vi "Process.vi"(8 "error in":errorcluster, 11 "demoForJoe":refnum<class "demoForJoe.lvclass">) -> (0 "error out":errorcluster, 3 "demoForJoe out":refnum<class "demoForJoe.lvclass">)   [LabVIEW 2016, in "demoForJoe.lvclass"]
doc: "---------------------------------------------------------------\nJKI State Machine Objects™\nhttp://jki.net/state-machine-objects/\nCopyright (C) 2005-2015, JKI <info@jki.net>\nALL RIGHTS RESERVED"
uses:
  demoForJoe.lvclass
  C:/Program Files (x86)/National Instruments/LabVIEW 2016/vi.lib/JKI/JKI SMO/SMO/SMO.lvclass
  Typedefs/PrivateEvents--demoForJoe.StringMethod.ctl
  <vilib>/JKI/JKI SMO/SMO/Typedefs/Parent Call--Enum.ctl
  <vilib>/JKI/JKI SMO/SMO/SMO.lvclass
panel:
  out "StringMethod":T1
  # "For instructions on how to use the JKI State Machine Objects, examples and video tutorials, visit:\nhttp://jki.net/state-machine-objects/\n\nJKI State Machine Objects™\nhttp://jki.net/state-machine-objects/\nCopyright (C) 2005-2015, JKI <info@jki.net>\nALL RIGHTS RESERVED"
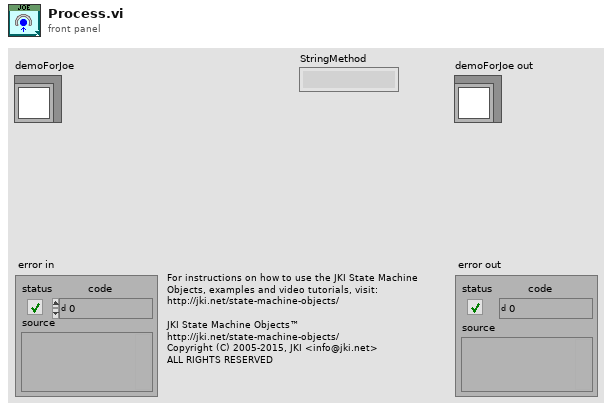
[diagram p1: front panel]
types:
  T1 = typedef "demoForJoe.lvclass/PrivateEvents--demoForJoe.StringMethod.ctl" = string
  T2 = typedef "SMO.lvclass/Parent Call--Enum.ctl" = enum16{"Allows parent to run", "Does not request parent to run"}
  T3 = enum32{"invalid app kind", "Development System", "Run Time System", "Student Edition", "Embedded LabVIEW", "Evaluation", "Custom"}
  T4 = enum32{"Invalid", "Standard", "Closed", "Hidden", "Minimized", "Maximized"}
  T5 = enum32{"Bad", "Idle", "Run top level", "Running"}
  T6 = cluster{"Core":cluster{"Current VI Reference":refnum<vi>, "Close Panel on Exit?":bool, "error":errorcluster}, "Self Reference":refnum<class "demoForJoe.lvclass">, "Your string data":string}
  T7 = cluster{"Current VI Reference":refnum<vi>, "Close Panel on Exit?":bool, "error":errorcluster}
  T8 = typedef "SMO.lvclass/Protected Events.ctl" = cluster{"StopProcesses":refnum<user-event>, "AbortProcesses":refnum<user-event>, "Config Changed":refnum<user-event>, "Dependency":refnum<user-event>}
  T9 = typedef "demoForJoe.lvclass/PrivateEvents--Cluster.ctl" = cluster{"StringMethod":refnum<user-event>}
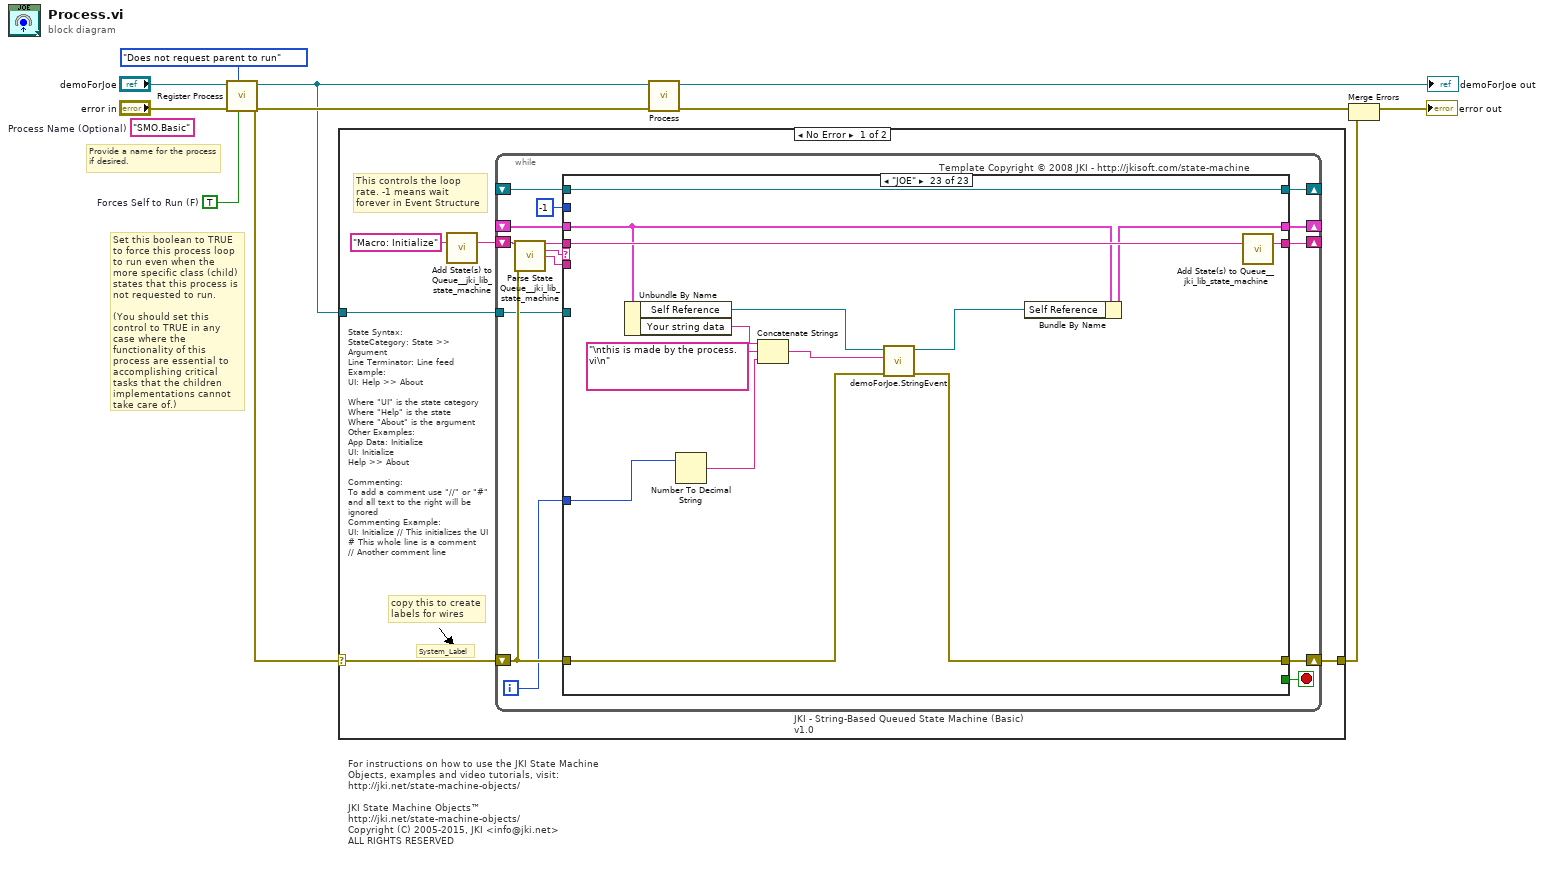
[diagram p0: block diagram]
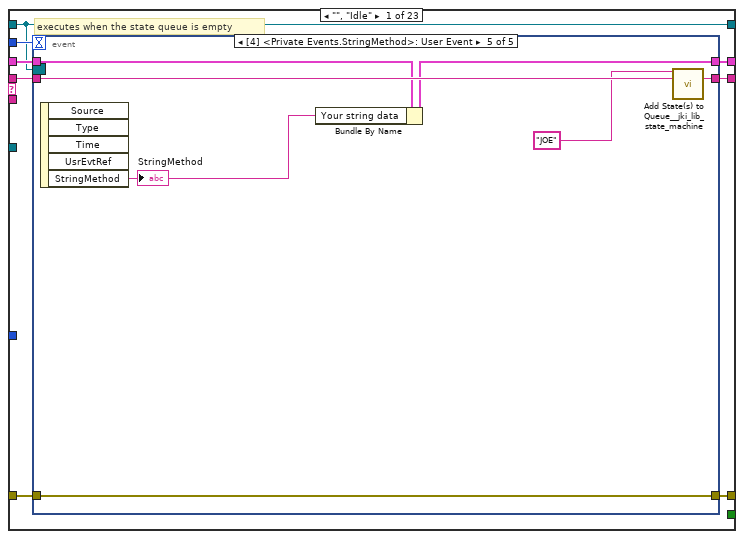
[diagram p2: hidden frame]
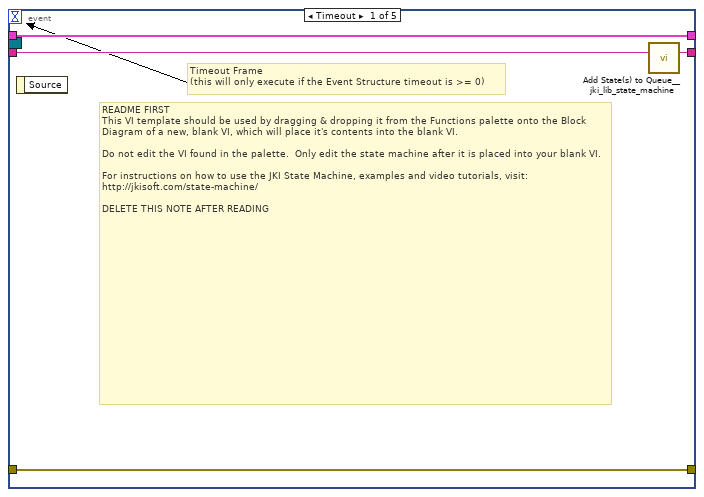
[diagram p3: hidden frame]
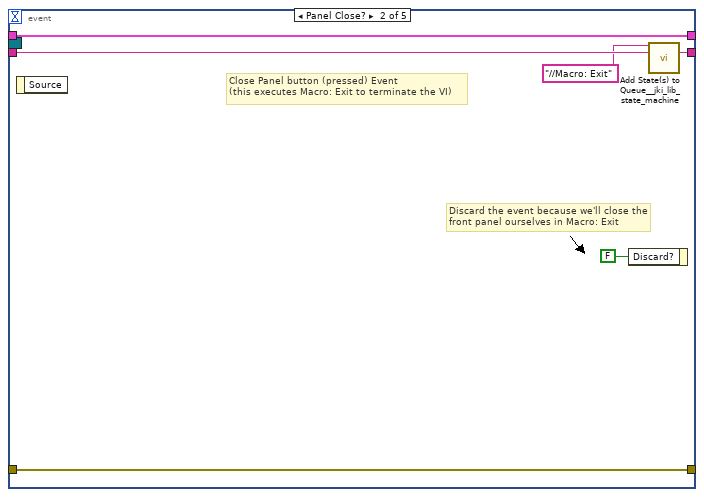
[diagram p4: hidden frame]
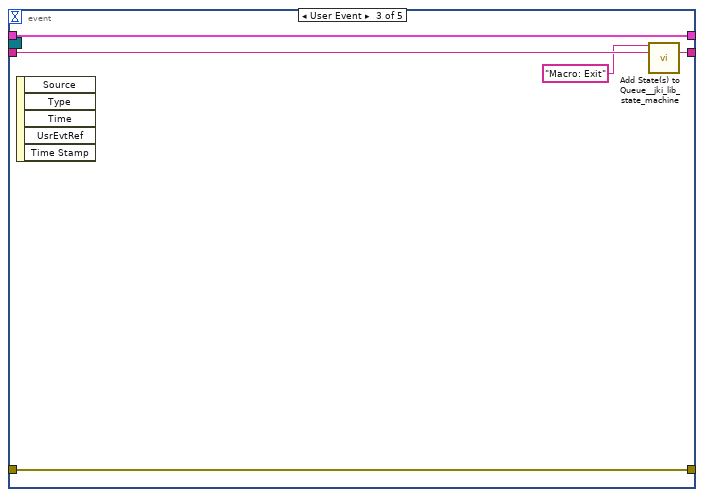
[diagram p5: hidden frame]
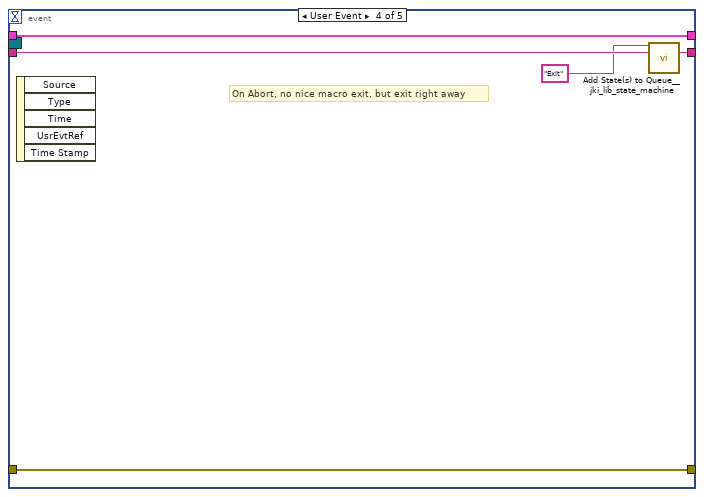
[diagram p6: hidden frame]
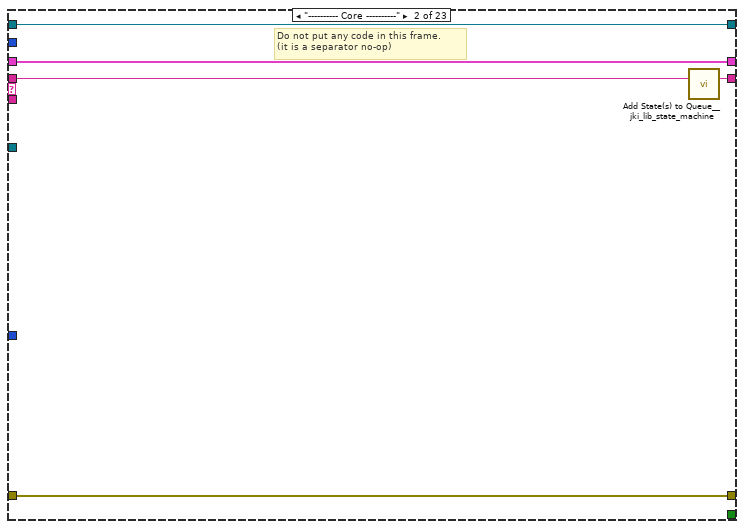
[diagram p7: hidden frame]
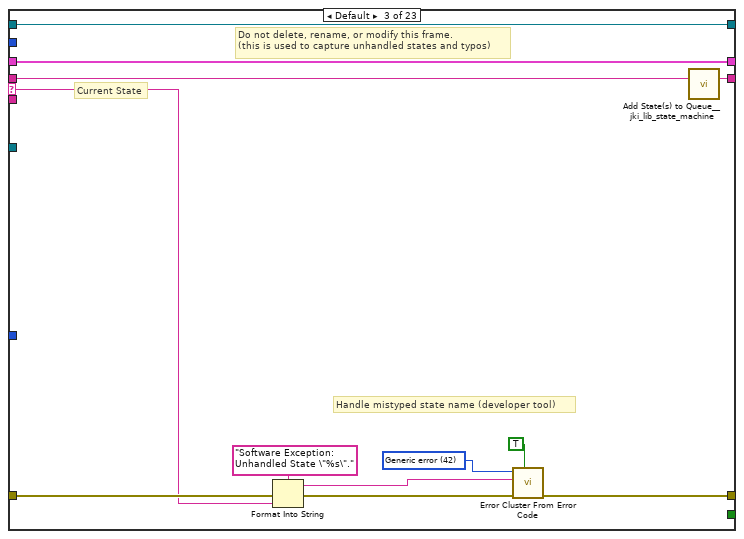
[diagram p8: hidden frame]
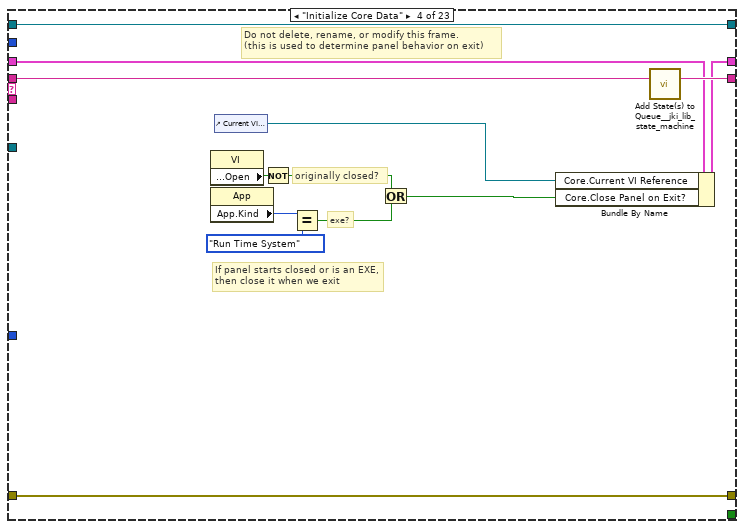
[diagram p9: hidden frame]
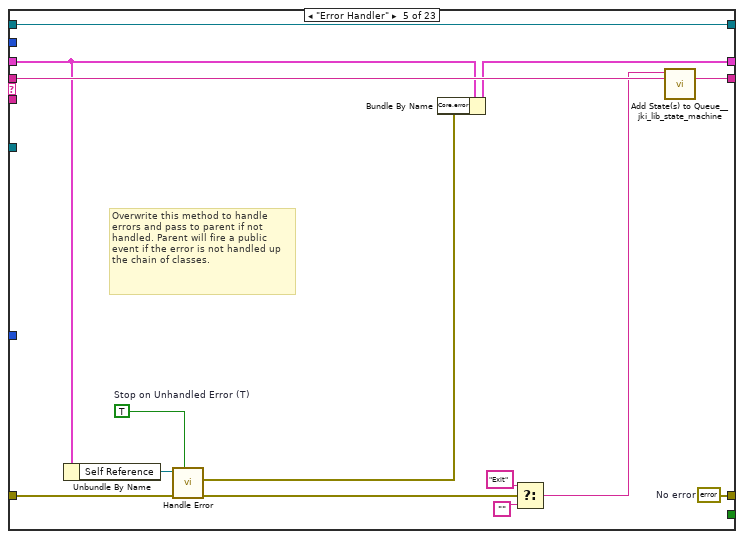
[diagram p10: hidden frame]
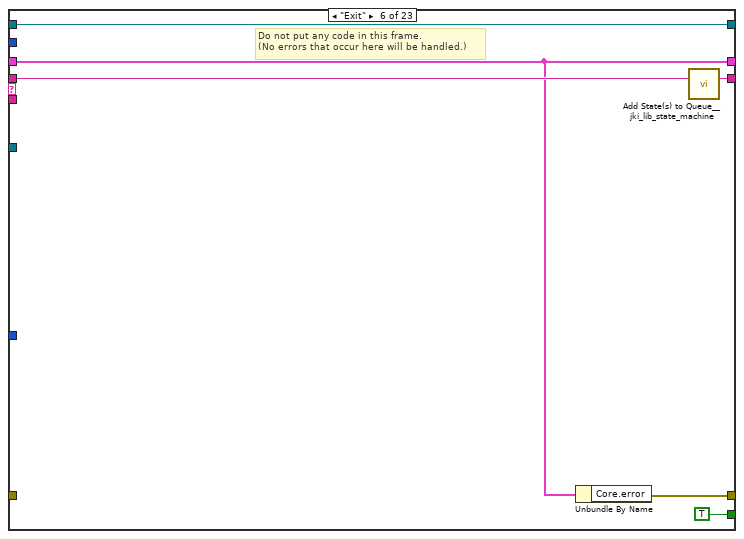
[diagram p11: hidden frame]
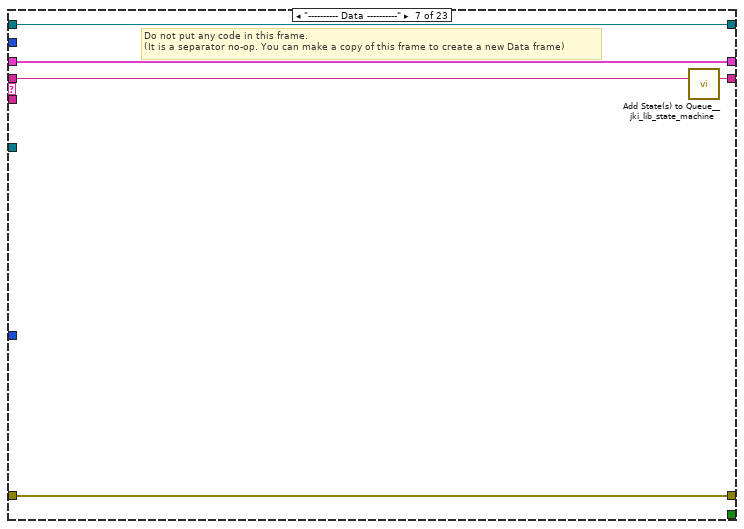
[diagram p12: hidden frame]
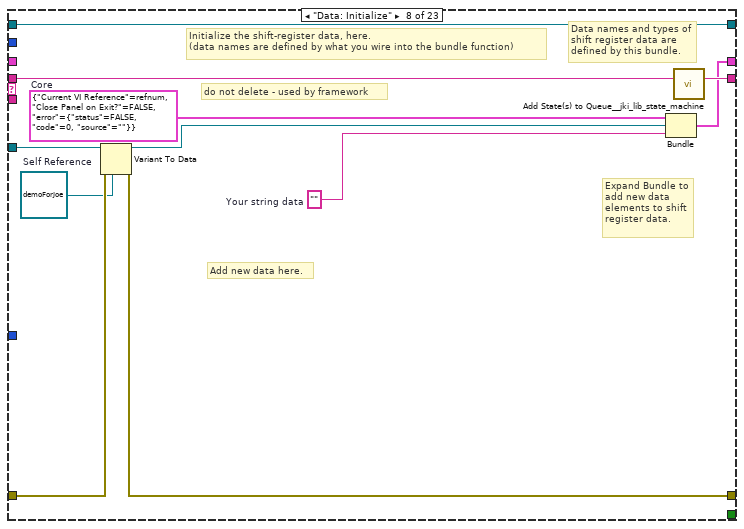
[diagram p13: hidden frame]
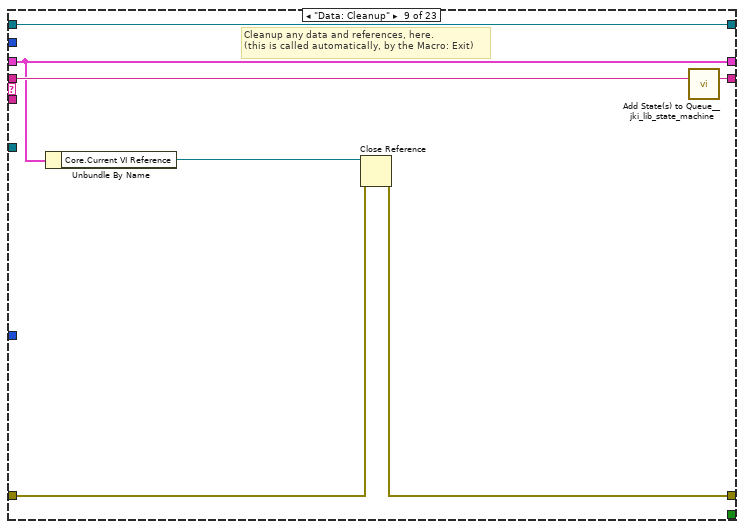
[diagram p14: hidden frame]
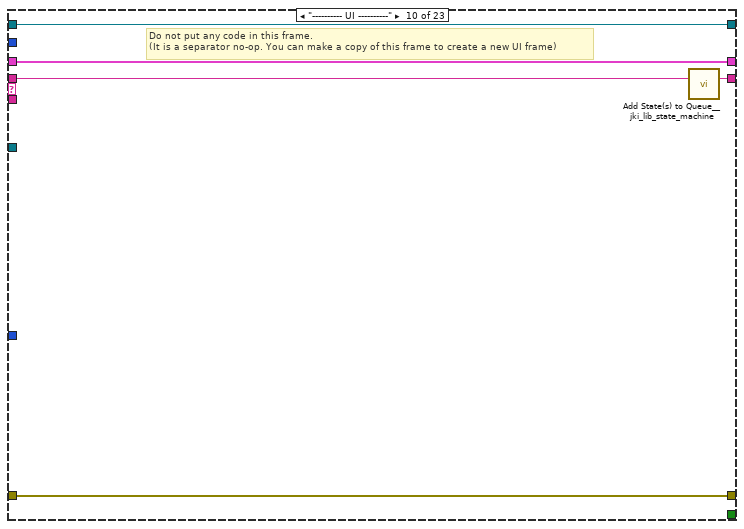
[diagram p15: hidden frame]
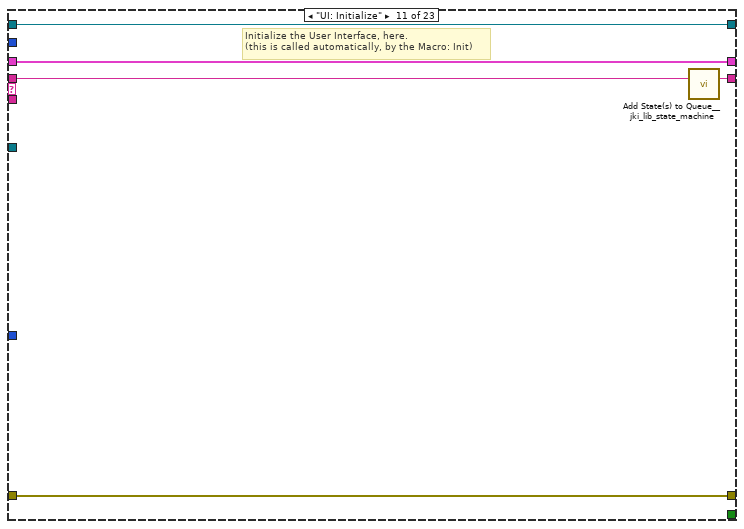
[diagram p16: hidden frame]
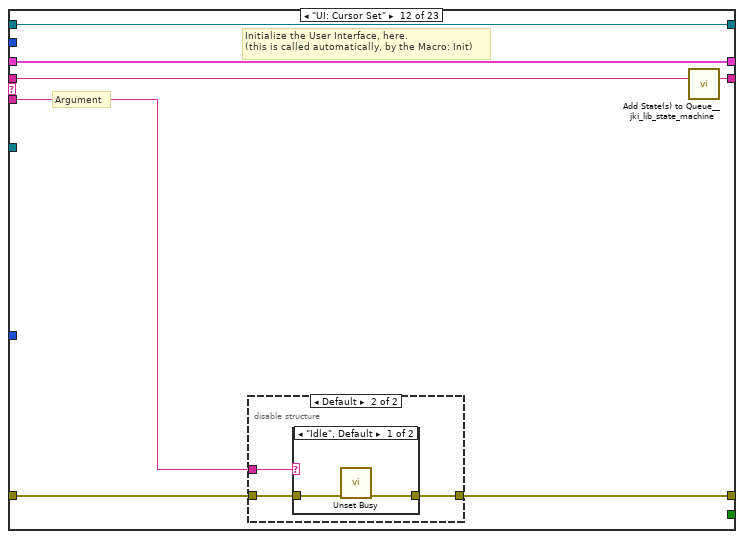
[diagram p17: hidden frame]
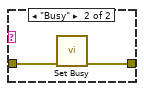
[diagram p19: hidden frame]
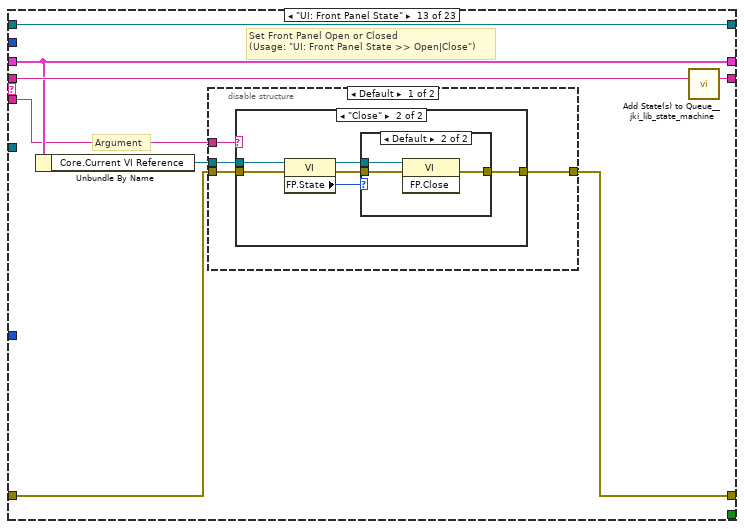
[diagram p20: hidden frame]
diagram:
  w1 = TRUE  # Forces Self to Run (F)
  (unwired) "SMO.Basic"  # Process Name (Optional)
  # "Provide a name for the process\nif desired."
  # "Set this boolean to TRUE to force this process loop to run even when the more specific class (child) states that this process is not requested to run.\n\n(You should set this control to TRUE in any case where the functionality of this process are essential to accomplishing critical tasks that the children implementations cannot take care of.)"
  # "For instructions on how to use the JKI State Machine Objects, examples and video tutorials, visit:\nhttp://jki.net/state-machine-objects/\n\nJKI State Machine Objects™\nhttp://jki.net/state-machine-objects/\nCopyright (C) 2005-2015, JKI <info@jki.net>\nALL RIGHTS RESERVED"
  n1 = call <vilib>:"Register Process.vi"("Forces Self to Run (F)"=w1, "Parent Call"=Parent_Call--Enum."Does not request parent to run", "error in (no error)"="error in", "SMO"="demoForJoe") -> ("error out"=w7:errorcluster, "SMO out"=w6:refnum<class "demoForJoe.lvclass">)  [unwired: 6 in]
  n2 = case shown="No Error" w7 {
    selector: w7 -> [w12 w291]
    tunnel: w6 -> [w13 _]
    tunnel: [w11 w291] -> w3
    frame No Error {
      # "State Syntax:\nStateCategory: State >> Argument\nLine Terminator: Line feed\nExample:\nUI: Help >> About\n\nWhere \"UI\" is the state category\nWhere \"Help\" is the state\nWhere \"About\" is the argument\nOther Examples:\nApp Data: Initialize\nUI: Initialize\nHelp >> About\n\nCommenting:\nTo add a comment use \"//\" or \"#\" and all text to the right will be ignored\nCommenting Example:\nUI: Initialize // This initializes the UI\n# This whole line is a comment\n// Another comment line"
      # "copy this to create labels for wires"
      # "This controls the loop rate. -1 means wait forever in Event Structure"
      # "System_Label"
      n3 = call <vilib>:"Add State(s) to Queue__jki_lib_state_machine.vi"("State(s) in (\"\")"="Macro: Initialize") -> ("States Out"=w15:string)  [unwired: 14 in]
      n4 = while "JKI - String-Based Queued State Machine (Basic) v1.0" {
        shift-right: [w23] -> _
        shift-left: _ -> [w22]
        shift-right: [w26] -> w11
        shift-left: w12 -> [w20]
        shift-right: [w25] -> _
        shift-left: w15 -> [w27]
        tunnel: w13 -> [w19]
        shift-right: [w18] -> _
        shift-left: _ -> [w17]
        i -> [w16]
        stop <- w24 stop-if-true
        # "Template Copyright © 2008 JKI - http://jkisoft.com/state-machine"
        n5 = call <vilib>:"Parse State Queue__jki_lib_state_machine.vi"("State Queue"=w27, "Error In (no error)"=w20) -> ("Remaining States"=w29:string, "Current State"=w30:string, "Arguments"=w28:string)  [unwired: 11 in]
        n6 = case shown="\"JOE\"" w30 {
          selector: w30 -> [_ _ w72 _ _ _ _ _ _ _ _ _ _ _ _ _ _ _ _ _ _ _ _]
          tunnel: w29 -> [w38 w70 w76 w95 w109 w115 w120 w131 w138 w143 w148 w155 w171 w203 w217 w231 w236 w247 w252 w265 w271 w276 w290]
          tunnel: w28 -> [_ _ _ _ _ _ _ _ _ _ _ w149 w165 _ _ _ _ _ _ _ _ _ _]
          tunnel: w22 -> [w36 w67 w74 w86 w103 w111 w117 _ w133 w140 w146 w153 w167 w200 w213 w222 w233 w244 w249 w263 w269 w274 w287]
          tunnel: [w35 w68 w78 w92 w104 w110 w118 w126 w134 w141 w145 w150 w168 w201 w215 w229 w234 w238 w250 w258 w267 w272 w282] -> w26
          tunnel: w20 -> [w34 w68 w77 w92 w105 _ w118 w127 w135 w141 w145 w151 w169 w201 w215 w229 w234 w239 w250 w259 w267 w272 w283]
          tunnel: [w37 w69 w75 w94 w108 w114 w119 w130 w137 w142 w147 w154 w170 w202 w216 w230 w235 w246 w251 w264 w270 w275 w289] -> w25
          tunnel: [_ _ _ _ _ TRUE _ _ _ _ _ _ _ _ _ _ _ _ _ _ _ _ _] -> w24
          tunnel: [w33 w67 w74 w93 w102 w111 w117 w129 w133 w140 w146 w153 w167 w200 w213 w222 w233 w244 w249 w263 w269 w274 w286] -> w23
          tunnel: -1 ("Timeout") -> [w32 _ _ _ _ _ _ _ _ _ _ _ _ _ _ _ _ _ _ _ _ _ _]
          tunnel: w19 -> [_ _ _ _ _ _ _ w124 _ _ _ _ _ _ _ _ _ _ _ _ _ _ _]
          tunnel: [w31 w66 w71 w83 w107 w112 w116 w122 w132 w139 w144 w152 w164 w199 w214 w223 w232 w245 w248 w262 w268 w273 w288] -> w18
          tunnel: w17 -> [w31 w66 w71 w83 w107 w112 w116 w122 w132 w139 w144 w152 w164 w199 w214 w223 w232 w245 w248 _ w268 w273 w288]
          tunnel: w16 -> [_ _ _ _ _ _ _ _ _ _ _ _ _ _ _ _ _ _ _ _ _ _ w278]
          frame "", "Idle" {
            # "executes when the state queue is empty"
            n7 = event shown="[4] <Private Events.StringMethod>: User Event" {
              selector: w31 -> [_ _ _ _ _]
              dyn-events: _ -> [_ _ _ _ _]
              timeout: w32 -> [_ _ _ _ _]
              tunnel: w38 -> [w42 w48 w53 w58 w65]
              tunnel: [w41 w47 w52 w57 w64] -> w37
              tunnel: w36 -> [w40 w45 w50 w55 w61]
              tunnel: [w39 w46 w51 w56 w63] -> w35
              tunnel: w34 -> [w39 w46 w51 w56 w63]
              tunnel: [w40 w45 w50 w55 w59] -> w33
              event Timeout {
                # "README FIRST\nThis VI template should be used by dragging & dropping it from the Functions palette onto the Block Diagram of a new, blank VI, which will place it's contents into the blank VI.\n\nDo not edit the VI found in the palette.  Only edit the state machine after it is placed into your blank VI.\n\nFor instructions on how to use the JKI State Machine, examples and video tutorials, visit:\nhttp://jkisoft.com/state-machine/\n\nDELETE THIS NOTE AFTER READING"
                # "Timeout Frame\n(this will only execute if the Event Structure timeout is >= 0)"
                n8 = event-data() -> ()  [unwired: 1 in, 1 out]
                n9 = call <vilib>:"Add State(s) to Queue__jki_lib_state_machine.vi"("State(s) in (\"\")"=w42) -> ("States Out"=w41:string)  [unwired: 14 in]
              }
              event Panel Close? {
                # "Discard the event because we'll close the front panel ourselves in Macro: Exit"
                # "Close Panel button (pressed) Event\n(this executes Macro: Exit to terminate the VI)"
                n10 = event-data() -> ()  [unwired: 1 in, 1 out]
                n11 = event-data("Discard?"=FALSE) -> ()  [unwired: 1 in, 1 out]
                n12 = call <vilib>:"Add State(s) to Queue__jki_lib_state_machine.vi"("State(s) in Front (\"\")"="//Macro: Exit", "State(s) in (\"\")"=w48) -> ("States Out"=w47:string)  [unwired: 13 in]
              }
              event User Event {
                n13 = event-data() -> ()  [unwired: 1 in, 5 out]
                n14 = call <vilib>:"Add State(s) to Queue__jki_lib_state_machine.vi"("State(s) in Front (\"\")"="Macro: Exit", "State(s) in (\"\")"=w53) -> ("States Out"=w52:string)  [unwired: 13 in]
              }
              event User Event {
                # "On Abort, no nice macro exit, but exit right away"
                n15 = event-data() -> ()  [unwired: 1 in, 5 out]
                n16 = call <vilib>:"Add State(s) to Queue__jki_lib_state_machine.vi"("State(s) in Front (\"\")"="Exit", "State(s) in (\"\")"=w58) -> ("States Out"=w57:string)  [unwired: 13 in]
              }
              event User Event {
                n17 = event-data() -> ("StringMethod"=w60:T1)  [unwired: 1 in, 4 out]
                "StringMethod" <- w60
                n18 = Bundle By Name(cluster=w61, "Your string data"=w60) -> (w59:T6)
                n19 = call <vilib>:"Add State(s) to Queue__jki_lib_state_machine.vi"("State(s) in Front (\"\")"="JOE" ("State(s) in Front (\"\")"), "State(s) in (\"\")"=w65) -> ("States Out"=w64:string)  [unwired: 13 in]
              }
            }
          }
          frame "---------- Core ----------" {
            # "Do not put any code in this frame.\n(it is a separator no-op)"
            n20 = call <vilib>:"Add State(s) to Queue__jki_lib_state_machine.vi"("State(s) in (\"\")"=w70) -> ("States Out"=w69:string)  [unwired: 14 in]
          }
          frame Default {
            w81 = 42 items=["No error", "Argument error", "Memory is full", "Out of zone", "End of file", "File already open", "Generic file I/O error", "File not found", "File permission error", "Disk is full", "Duplicate path", "Too many files open", "System feature not enabled", "Resource file not found", "Cannot add resource", "Resource not found", "Image not found", "Image memory error", "Pen does not exist", "Config type invalid", "Config token not found", "Config parse error", "Config memory error", "Bad external code format", "Bad external code offset", "External code not present", "Null window", "Destroy window error", "Null menu", "Print aborted", "Bad print record", "Print driver error", "Windows error during printing", "Memory error during printing", "Print dialog error", "Generic print error", "Invalid device refnum", "Device not found", "Device parameter error", "Device unit error", "Cannot open device", "Device call aborted", "Generic error", "Cancelled by user", "Object ID too low", "Object ID too high", "Object not in heap", "Unknown heap", "Unknown object (invalid DefProc)", "Unknown object (DefProc not in table)", "Message out of range", "Invalid (null) method", "Unknown message", "Manager call not supported", "Bad address", "Network operation in progress", "Network operation timed out", "Connection is busy", "Network attribute not supported", "Network error", "Address in use", "System out of memory", "Connection aborted", "Connection refused", "Not connected", "Already connected", "Connection closed", "Initialization error (interapplication manager)", "Bad occurrence", "Wait on unbound occurrence handler", "Occurrence queue overflow", "Datalog type conflict", "Unused", "Unrecognized type (interapplication manager)", "Memory corrupt", "Failed to make temporary DLL", "Old CIN version", "Drag socket not found", "Failed to load drop-object", "Failed to register OLE object", "Failed to release OLE object", "Format specifier type mismatch", "Unknown format specifier", "Too few format specifiers", "Too many format specifiers", "Scan failed", "Newer CIN version", "Error converting to variant", "Runtime menu error", "Password tampered", "Variant attribute not found", "Incompatible variant data type", "Event data is not available", "Event Store is not present", "Occurrence is not found", "Event Queue is not created", "Event info is not available", "Refnum passed is NULL", "Error retrieving Class GUID", "Error retrieving CoClass GUID", "Error retrieving TypeLib GUID.", "Bad built application magic bytes.", "Specific driver is different from the specific driver associated with the Logical Name.", "There is no session opened to the class driver.", "Max Error", "MAX - Error with config objects", "MAX - Error loading configuration", "MAX - Group not supported"]
            # "Current State"
            # "Do not delete, rename, or modify this frame.\n(this is used to capture unhandled states and typos)"
            # "Handle mistyped state name (developer tool)"
            n21 = Format Into String(format string="Software Exception: Unhandled State \"%s\"." ("message"), error in=w77, w72) -> (resulting string=w80:string, error out=w79:errorcluster)  [unwired: 1 in]
            n22 = call <vilib>:"Error Cluster From Error Code.vi"("show call chain? (False)"=TRUE, "error in (no error)"=w79, "error message (\"\")"=w80, "error code (0)"=w81) -> ("error out"=w78:errorcluster)  [unwired: 5 in]
            n23 = call <vilib>:"Add State(s) to Queue__jki_lib_state_machine.vi"("State(s) in (\"\")"=w76) -> ("States Out"=w75:string)  [unwired: 14 in]
          }
          frame "Initialize Core Data" {
            # "Do not delete, rename, or modify this frame.\n(this is used to determine panel behavior on exit)"
            # "originally closed?"
            # "exe?"
            # "If panel starts closed or is an EXE, then close it when we exit"
            n24 = property class="VI"() -> ("Front Panel.Open"=w91:bool)  [unwired: 2 in, 2 out]
            n25 = property class="App"() -> ("App.Kind"=w90:T3)  [unwired: 2 in, 2 out]
            n26 = control-ref of="Current VI Reference"() -> (w84:refnum<vi>)
            n27 = Not(x=w91) -> (.not. x?=w88:bool)
            n28 = Equal?(x=w90, y=T3."Run Time System" ("Application:Kind")) -> (x = y?=w87:bool)
            n29 = Or(x=w88, y=w87) -> (x .or. y?=w85:bool)
            n30 = Bundle By Name(cluster=w86, "Core.Current VI Reference"=w84, "Core.Close Panel on Exit?"=w85) -> (w93:T6)
            n31 = call <vilib>:"Add State(s) to Queue__jki_lib_state_machine.vi"("State(s) in (\"\")"=w95) -> ("States Out"=w94:string)  [unwired: 14 in]
          }
          frame "Error Handler" {
            w96 = TRUE  # Stop on Unhandled Error (T)
            w104 = errorcluster {"status"=FALSE, "code"=0, "source"=""}  # No error
            # "Overwrite this method to handle errors and pass to parent if not handled. Parent will fire a public event if the error is not handled up the chain of classes."
            n32 = Unbundle By Name(w103) -> ("Self Reference"=w106:refnum<class "demoForJoe.lvclass">)
            n33 = call-dynamic "Handle Error.vi"("Stop on Unhandled Error (T)"=w96, "error in"=w105, "SMO"=w106) -> ("handling error"=w97:errorcluster, "Unhandled error"=w100:errorcluster)  [unwired: 6 in, 1 out]
            n34 = Bundle By Name(cluster=w103, "Core.error"=w100) -> (w102:T6)
            n35 = Select(t="Exit", s=w97, f="") -> (s? t:f=w101:string)
            n36 = call <vilib>:"Add State(s) to Queue__jki_lib_state_machine.vi"("State(s) in Front (\"\")"=w101, "State(s) in (\"\")"=w109) -> ("States Out"=w108:string)  [unwired: 13 in]
          }
          frame "Exit" {
            # "Do not put any code in this frame.\n(No errors that occur here will be handled.)"
            n37 = Unbundle By Name(w111) -> ("Core.error"=w110:errorcluster)
            n38 = call <vilib>:"Add State(s) to Queue__jki_lib_state_machine.vi"("State(s) in (\"\")"=w115) -> ("States Out"=w114:string)  [unwired: 14 in]
          }
          frame "---------- Data ----------" {
            # "Do not put any code in this frame.\n(It is a separator no-op. You can make a copy of this frame to create a new Data frame)"
            n39 = call <vilib>:"Add State(s) to Queue__jki_lib_state_machine.vi"("State(s) in (\"\")"=w120) -> ("States Out"=w119:string)  [unwired: 14 in]
          }
          frame "Data: Initialize" {
            w121 = T7 {"Current VI Reference"=refnum, "Close Panel on Exit?"=FALSE, "error"={"status"=FALSE, "code"=0, "source"=""}}  # Core
            w125 = refnum<class "demoForJoe.lvclass"> refnum  # Self Reference
            w128 = ""  # Your string data
            # "do not delete - used by framework"
            # "Expand Bundle to add new data elements to shift register data."
            # "Add new data here."
            # "Data names and types of shift register data are defined by this bundle."
            # "Initialize the shift-register data, here.\n(data names are defined by what you wire into the bundle function)"
            n40 = Variant To Data(error in=w127, type=w125, Variant=w124) -> (data=w123:refnum<class "demoForJoe.lvclass">, error out=w126:errorcluster)
            n41 = Bundle("Core"=w121, "Self Reference"=w123, "Your string data"=w128) -> (w129:T6)  [unwired: 1 in]
            n42 = call <vilib>:"Add State(s) to Queue__jki_lib_state_machine.vi"("State(s) in (\"\")"=w131) -> ("States Out"=w130:string)  [unwired: 14 in]
          }
          frame "Data: Cleanup" {
            # "Cleanup any data and references, here.\n(this is called automatically, by the Macro: Exit)"
            n43 = Unbundle By Name(w133) -> ("Core.Current VI Reference"=w136:refnum<vi>)
            n44 = Close Reference(reference=w136, error in (no error)=w135) -> (error out=w134:errorcluster)
            n45 = call <vilib>:"Add State(s) to Queue__jki_lib_state_machine.vi"("State(s) in (\"\")"=w138) -> ("States Out"=w137:string)  [unwired: 14 in]
          }
          frame "---------- UI ----------" {
            # "Do not put any code in this frame.\n(It is a separator no-op. You can make a copy of this frame to create a new UI frame)"
            n46 = call <vilib>:"Add State(s) to Queue__jki_lib_state_machine.vi"("State(s) in (\"\")"=w143) -> ("States Out"=w142:string)  [unwired: 14 in]
          }
          frame "UI: Initialize" {
            # "Initialize the User Interface, here.\n(this is called automatically, by the Macro: Init)"
            n47 = call <vilib>:"Add State(s) to Queue__jki_lib_state_machine.vi"("State(s) in (\"\")"=w148) -> ("States Out"=w147:string)  [unwired: 14 in]
          }
          frame "UI: Cursor Set" {
            # "Argument"
            # "Initialize the User Interface, here.\n(this is called automatically, by the Macro: Init)"
            n48 = disable-structure shown="Default" {
              disable-tunnel: w151 -> [w156 w159]
              disable-tunnel: [w156 w158] -> w150
              disable-tunnel: w149 -> [_ w157]
              frame condition #0 {
              }
              frame condition #1 (active) {
                n49 = case shown="\"Idle\", Default" w157 {
                  tunnel: w159 -> [w161 w163]
                  tunnel: [w160 w162] -> w158
                  frame "Idle", Default {
                    n50 = call <vilib>:"Unset Busy.vi"("error in (no error)"=w161) -> ("error out"=w160:errorcluster)  [unwired: 10 in]
                  }
                  frame "Busy" {
                    n51 = call <vilib>:"Set Busy.vi"("error in (no error)"=w163) -> ("error out"=w162:errorcluster)  [unwired: 9 in, 1 out]
                  }
                }
              }
            }
            n52 = call <vilib>:"Add State(s) to Queue__jki_lib_state_machine.vi"("State(s) in (\"\")"=w155) -> ("States Out"=w154:string)  [unwired: 14 in]
          }
          frame "UI: Front Panel State" {
            # "Argument"
            # "Set Front Panel Open or Closed\n(Usage: \"UI: Front Panel State >> Open|Close\")"
            n53 = Unbundle By Name(w167) -> ("Core.Current VI Reference"=w166:refnum<vi>)
            n54 = disable-structure shown="Default" {
              disable-tunnel: w169 -> [w175 w198]
              disable-tunnel: [w174 w198] -> w168
              disable-tunnel: w166 -> [w173 _]
              disable-tunnel: w165 -> [w172 _]
              frame condition #0 (active) {
                n55 = case shown="\"Close\"" w172 {
                  tunnel: w175 -> [w179 w192]
                  tunnel: [w181 w193] -> w174
                  tunnel: w173 -> [w180 w190]
                  frame "Open", Default {
                    n56 = property class="VI"(reference=w180, error in=w179) -> (reference out=w177:refnum<vi>, error out=w178:errorcluster, "FP.State"=w176:T4)
                    n57 = case shown="\"Closed\"" w176 {
                      tunnel: [w184 w187] -> w181
                      tunnel: w178 -> [w183 w187]
                      tunnel: w177 -> [w182 _]
                      frame "Closed" {
                        n58 = invoke class="VI" method="FP.Open"(reference=w182, error in=w183, "Activate"=TRUE, "State"=T4."Standard") -> (error out=w184:errorcluster)  [unwired: 1 in, 4 out]
                      }
                      frame Default {
                      }
                    }
                  }
                  frame "Close" {
                    n59 = property class="VI"(reference=w190, error in=w192) -> (reference out=w189:refnum<vi>, error out=w191:errorcluster, "FP.State"=w188:T4)
                    n60 = case shown="Default" w188 {
                      tunnel: [w194 w197] -> w193
                      tunnel: w191 -> [w194 w196]
                      tunnel: w189 -> [_ w195]
                      frame "Invalid", "Closed" {
                      }
                      frame Default {
                        n61 = invoke class="VI" method="FP.Close"(reference=w195, error in=w196) -> (error out=w197:errorcluster)  [unwired: 1 in, 2 out]
                      }
                    }
                  }
                }
              }
              frame condition #1 {
              }
            }
            n62 = call <vilib>:"Add State(s) to Queue__jki_lib_state_machine.vi"("State(s) in (\"\")"=w171) -> ("States Out"=w170:string)  [unwired: 14 in]
          }
          frame "---------- Macro ----------" {
            # "Do not put any code in this frame.\n(It is a separator no-op. You can make a copy of this frame to create a new Macro frame)"
            n63 = call <vilib>:"Add State(s) to Queue__jki_lib_state_machine.vi"("State(s) in (\"\")"=w203) -> ("States Out"=w202:string)  [unwired: 14 in]
          }
          frame "Macro: Initialize" {
            w208 = "UI: Initialize\nUI: Front Panel State >> Open"  # UI: Initialize UI: Front Panel State >> Open
            w204 = "Process: Sync"
            # "Initialization Macro\n(This is called once, when the VI starts)"
            n64 = control-ref of="This VI"() -> (w206:refnum<vi>)
            n65 = property class="VI"(reference=w206) -> ("Exec.State"=w205:T5)  [unwired: 1 in, 2 out]
            n66 = Equal?(x=w205, y=T5."Run top level") -> (x = y?=w211:bool)
            n67 = Select(t=w204, s=w211, f="") -> ()  [unwired: 1 out]
            n68 = call <vilib>:"Add State(s) to Queue__jki_lib_state_machine.vi"("State(s) in Front (\"\")"="Data: Initialize\nInitialize Core Data\nEvents: Register", "State(s) in (\"\")"=w204, "State(s) at Back (\"\")"=w208) -> ("States Out"=w207:string)  [unwired: 12 in]
            n69 = call <vilib>:"Add State(s) to Queue__jki_lib_state_machine.vi"("State(s) in Front (\"\")"=w207, "State(s) in (\"\")"=w217) -> ("States Out"=w216:string)  [unwired: 13 in]
          }
          frame "Macro: Exit" {
            # "Exit Macro\n(This is called once, when the VI exits)"
            n70 = Unbundle By Name(w222) -> ("Core.Close Panel on Exit?"=w228:bool)
            n71 = Select(t="UI: Front Panel State >> Close", s=w228, f="") -> (s? t:f=w225:string)
            n72 = call <vilib>:"Add State(s) to Queue__jki_lib_state_machine.vi"("State(s) in Front (\"\")"="Data: Cleanup\nEvents: Unregister", "State(s) in (\"\")"="Process: Sync", "State(s) at Back (\"\")"="Exit") -> ("States Out"=w219:string)  [unwired: 12 in]
            n73 = call <vilib>:"Add State(s) to Queue__jki_lib_state_machine.vi"("State(s) in (\"\")"=w225, "State(s) at Back (\"\")"=w219) -> ("States Out"=w224:string)  [unwired: 13 in]
            n74 = call <vilib>:"Add State(s) to Queue__jki_lib_state_machine.vi"("State(s) in Front (\"\")"=w224, "State(s) in (\"\")"=w231) -> ("States Out"=w230:string)  [unwired: 13 in]
          }
          frame "---------- Process ----------" {
            # "Template Separator\n(You can make a copy of, or modify, this frame)"
            n75 = call <vilib>:"Add State(s) to Queue__jki_lib_state_machine.vi"("State(s) in (\"\")"=w236) -> ("States Out"=w235:string)  [unwired: 14 in]
          }
          frame "Process: Sync" {
            n76 = Unbundle By Name(w244) -> ("Self Reference"=w240:refnum<class "demoForJoe.lvclass">)
            n77 = call <vilib>:"WaitOnProcessSync.vi"("error in (no error)"=w239, "SMO"=w240) -> ("error out"=w238:errorcluster, "Don't run?"=w243:bool)  [unwired: 7 in, 1 out]
            n78 = Select(t="Data: Cleanup\nEvents: Unregister\nExit", s=w243, f="") -> (s? t:f=w237:string)
            n79 = call <vilib>:"Add State(s) to Queue__jki_lib_state_machine.vi"("State(s) in Front (\"\")"=w237, "State(s) in (\"\")"=w247) -> ("States Out"=w246:string)  [unwired: 13 in]
          }
          frame "---------- Events ----------" {
            # "Template Separator\n(You can make a copy of, or modify, this frame)"
            n80 = call <vilib>:"Add State(s) to Queue__jki_lib_state_machine.vi"("State(s) in (\"\")"=w252) -> ("States Out"=w251:string)  [unwired: 14 in]
          }
          frame "Events: Register" {
            # "Expand to add\nmore events"
            n81 = Unbundle By Name(w263) -> ("Self Reference"=w260:refnum<class "demoForJoe.lvclass">)
            n82 = call <vilib>:"GetProtectedEvents.vi"("SMO"=w260) -> ("error out"=w254:errorcluster, "SMO Protected Events"=w261:T8, "SMO out"=w256:refnum<class "demoForJoe.lvclass">)  [unwired: 8 in]
            n83 = call "demoForJoe.GetPrivateEvents.vi"("error in (no error)"=w254, "demoForJoe"=w256) -> ("error out"=w253:errorcluster, "Private Events"=w255:T9)  [unwired: 7 in, 1 out]
            n84 = register-events(w261, w255) -> (reference out=w262:refnum<event-registration>, error out=w257:errorcluster)  [unwired: 2 in]
            n85 = Merge Errors(w259, w257, w253) -> (w258:errorcluster)
            n86 = call <vilib>:"Add State(s) to Queue__jki_lib_state_machine.vi"("State(s) in (\"\")"=w265) -> ("States Out"=w264:string)  [unwired: 14 in]
          }
          frame "Events: Unregister" {
            n87 = Unregister For Events(event registration refnum=w268, error in=w267) -> (error out=w266:errorcluster)
            n88 = call <vilib>:"Clear Errors.vi"("error in (no error)"=w266) -> ()  [unwired: 5 in, 2 out]
            n89 = call <vilib>:"Add State(s) to Queue__jki_lib_state_machine.vi"("State(s) in (\"\")"=w271) -> ("States Out"=w270:string)  [unwired: 14 in]
          }
          frame "---------- Action ----------" {
            n90 = call <vilib>:"Add State(s) to Queue__jki_lib_state_machine.vi"("State(s) in (\"\")"=w276) -> ("States Out"=w275:string)  [unwired: 14 in]
          }
          frame "JOE" {
            n91 = Unbundle By Name(w287) -> ("Self Reference"=w285:refnum<class "demoForJoe.lvclass">, "Your string data"=w281:string)
            n92 = Number To Decimal String(number=w278) -> (decimal integer string=w277:string)  [unwired: 1 in]
            n93 = Concatenate Strings(w281, "\nthis is made by the process.vi\n" ("string"), w277) -> (w279:string)
            n94 = call "demoForJoe.StringEvent.vi"("error in (no error)"=w283, "StringEvent"=w279, "demoForJoe"=w285) -> ("error out"=w282:errorcluster, "demoForJoe out"=w284:refnum<class "demoForJoe.lvclass">)  [unwired: 7 in]
            n95 = Bundle By Name(cluster=w287, "Self Reference"=w284) -> (w286:T6)
            n96 = call <vilib>:"Add State(s) to Queue__jki_lib_state_machine.vi"("State(s) in (\"\")"=w290) -> ("States Out"=w289:string)  [unwired: 14 in]
          }
        }
      }
    }
    frame Error {
    }
  }
  n97 = call-parent "Process.vi"("error in"=w7, "SMO"=w6) -> ("error out"=w4:errorcluster, "SMO out"=→"demoForJoe out":refnum<class "demoForJoe.lvclass">)  [unwired: 8 in]
  n98 = Merge Errors(w4, w3) -> (→"error out":errorcluster)
